vi "second.vi"() -> ()   [LabVIEW 2019]
panel:
  out "Meter":dbl(knob) scale=0.0..10.0
  in  "Slide":dbl(slide) scale=0.0..10.0
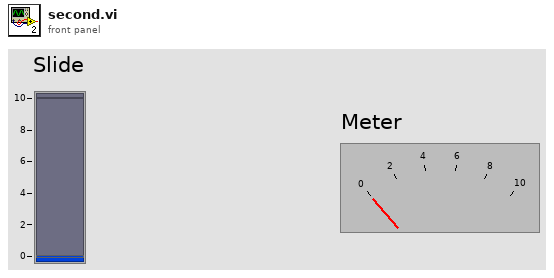
[diagram p1: front panel]
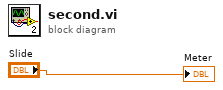
[diagram p0: block diagram]
diagram:
  "Meter" <- "Slide"
